vi "Global_WC_Drive_Encoder_Values.vi"() -> ()   [LabVIEW 2017]
panel:
  in  "Encoders":i32[](array[numeric])
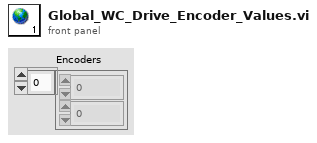
[diagram p1: front panel]
diagram:
